vi "Clean Imaging Data Address.vi"(9 "Imaging data displayed in":u32, 10 "Clean":bool, 11 "Imaging data address out":u32) -> (2 "Imaging data displayed in":u32, 3 "Imaging data address":u32)   [LabVIEW 2015]
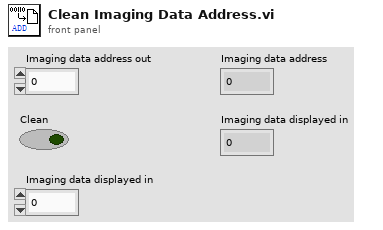
[diagram p1: front panel]
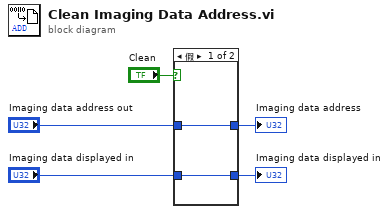
[diagram p0: block diagram]
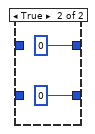
[diagram p2: hidden frame]
diagram:
  n1 = case shown="假" "Clean" {
    tunnel: "Imaging data address out" -> [w6 _]
    tunnel: "Imaging data displayed in" -> [w7 _]
    tunnel: [w6 u32 0 ("Imaging data address")] -> w4
    tunnel: [w7 u32 0 ("Imaging data displayed")] -> w5
    frame False {
    }
    frame True {
    }
  }
  "Imaging data displayed in" <- w5
  "Imaging data address" <- w4
